vi "String_Build String from Name Value Pairs.vi"(8 "Error":errorcluster, 9 "String Values":string[](array[string]), 10 "String Names":string[](array[string]), 11 "Start String":string) -> (0 "Error Out":errorcluster, 3 "String Out":string)   [LabVIEW 2020]
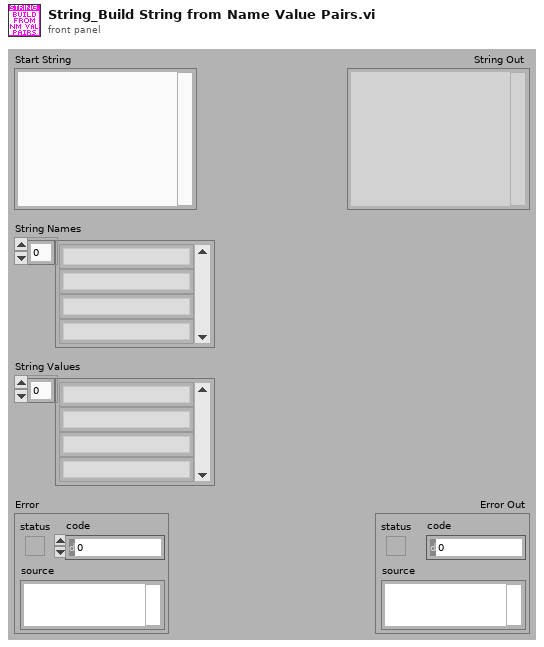
[diagram p1: front panel]
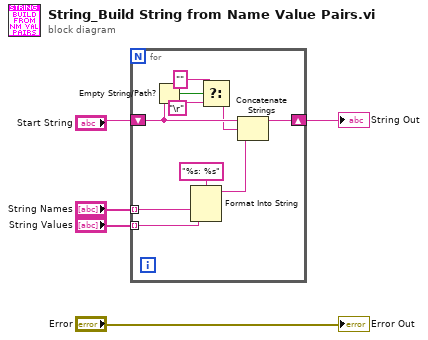
[diagram p0: block diagram]
diagram:
  n1 = for {
    tunnel: "String Names" -> [w14] mode=indexing
    tunnel: "String Values" -> [w13] mode=indexing
    shift-right: [w12] -> w2
    shift-left: "Start String" -> [w10]
    n2 = Empty String/Path?(string/path=w10) -> (empty?=w9:bool)
    n3 = Format Into String(format string="%s: %s", w14, w13) -> (resulting string=w11:string)  [unwired: 2 in, 1 out]
    n4 = Select(t="", s=w9, f="\r") -> (s? t:f=w7:string)
    n5 = Concatenate Strings(w10, w7, w11) -> (w12:string)
  }
  "String Out" <- w2
  "Error Out" <- "Error"
